vi "decodeTimeout.vi"(1 "reg_val":u16) -> (0 "timeout_mclks":u16)   [LabVIEW 2018]
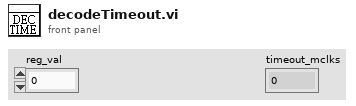
[diagram p1: front panel]
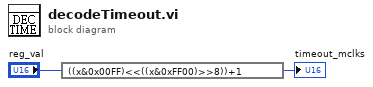
[diagram p0: block diagram]
diagram:
  n1 = expression code="((x&0x00FF)<<((x&0xFF00)>>8))+1"("reg_val") -> (→"timeout_mclks":u16)
